vi "测量流程.vi"(11 "控制命令":T1(ring)) -> ()   [LabVIEW 2016, in "斯坦道氨氮.lvlib"]
uses:
  <vilib>/ptbypt/NI_PtbyPt.lvlib
panel:
  out "x-y":dbl
  out "当前时间":timestamp
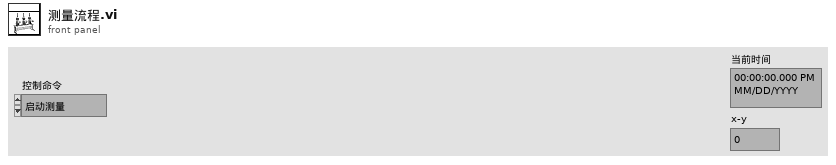
[diagram p1: front panel]
types:
  T1 = enum16{"启动测量", "标样核查", "零点核查", "跨度核查", "空白测试", "平行样测试", "加标回收", "空白校准", "标样校准", "初始化（清洗）", "停止测试", "仪器重启", "校时", "模式设置", "测量间隔设置"}
  T2 = cluster{"站号":u16, "量程切换":enum32{"H", "L", "AUTO"}, "控制命令":enum16{"启动测量", "标样核查", "零点核查", "跨度核查", "空白测试", "平行样测试", "加标回收", "空白校准", "标样校准", "初始化（清洗）", "停止测试", "仪器重启", "校时", "模式设置", "测量间隔设置"}, "模式设置":enum16{"待机", "连续模式", "周期模式", "定点模式", "受控模式", "手动模式"}, "测量间隔":u16}
  T3 = typedef "报警信息字段定义.ctl" = cluster{"时间":timestamp, "参数":string, "报警信息":string, "备注":string}
  T4 = cluster{"时间标识":timestamp, "设备":string, "日志信息":string, "流程参数":string}
  T5 = enum16{"空闲", "水样测试", "标样核查", "零点核查", "跨度核查", "空白测试", "平行样测试", "加标回收", "空白校准", "标样校准", "初始化（清洗）"}
  T6 = cluster{"系统时间":timestamp, "工作状态":u16, "测量模式":enum16{"待机", "连续模式", "周期模式", "定点模式", "受控模式", "手动模式"}, "告警代码":u16, "故障代码":u16, "日志代码":u16, "软件版本":u16, "F0":sgl, "F1":sgl, "F2":sgl, "F3":sgl, "T":sgl, "H":sgl, "id":u16, "flowid":u16, "量程":u16, "总磷控温温度1":sgl, "营养盐控温温度2":sgl, "ADC":sgl}
  T7 = cluster{"水样测试量程模式":enum16{"H", "L", "AUTO"}, "空白核查量程模式":enum16{"H", "L", "AUTO"}, "跨度核查量程模式":enum16{"H", "L", "AUTO"}, "加标回收量程模式":enum16{"H", "L", "AUTO"}, "标样核查量程模式":enum16{"H", "L", "AUTO"}}
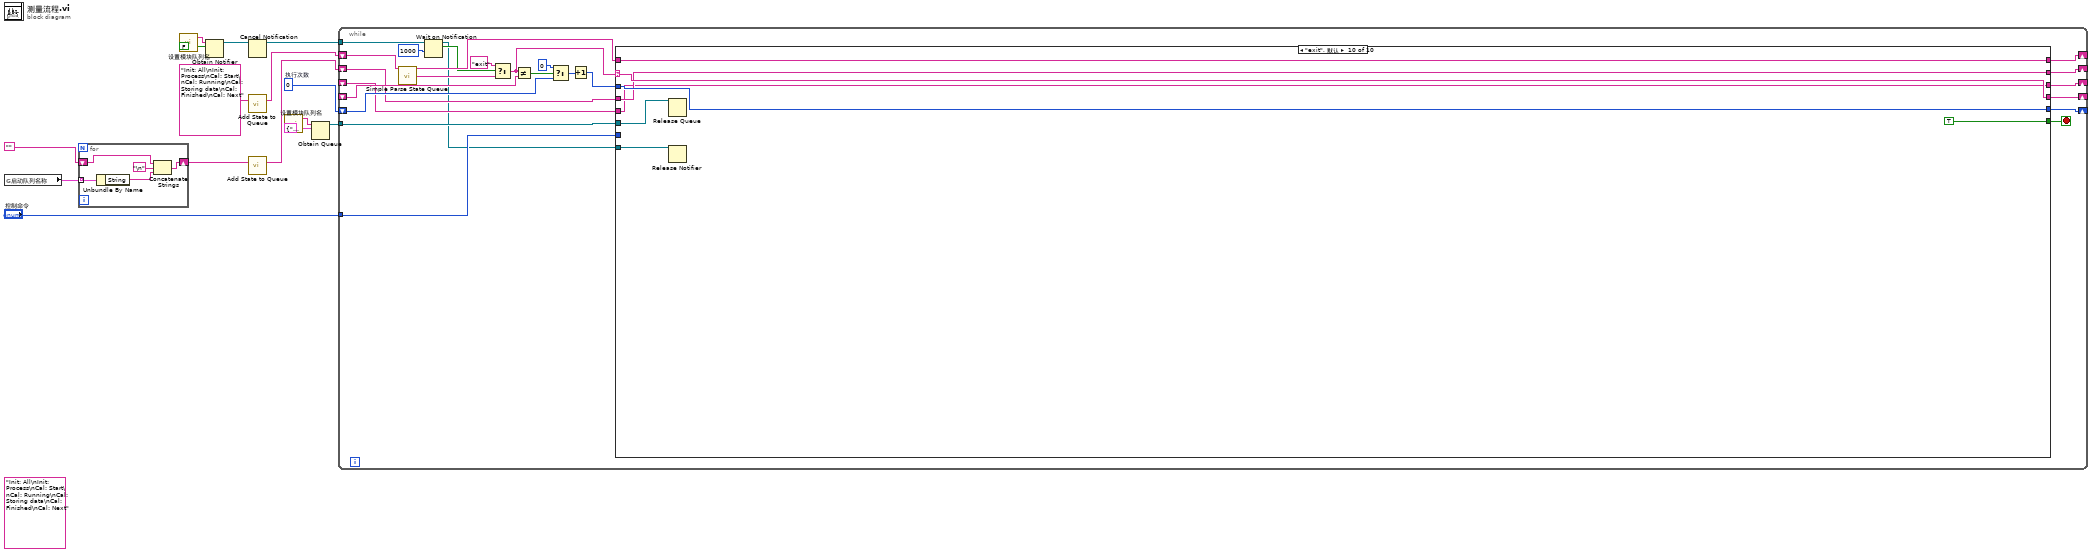
[diagram p0: block diagram]
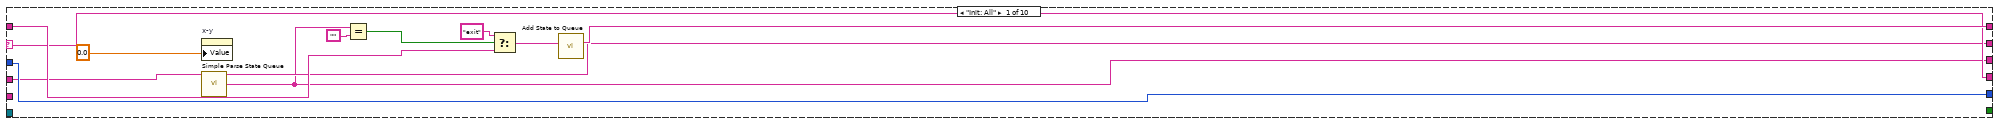
[diagram p2: hidden frame]
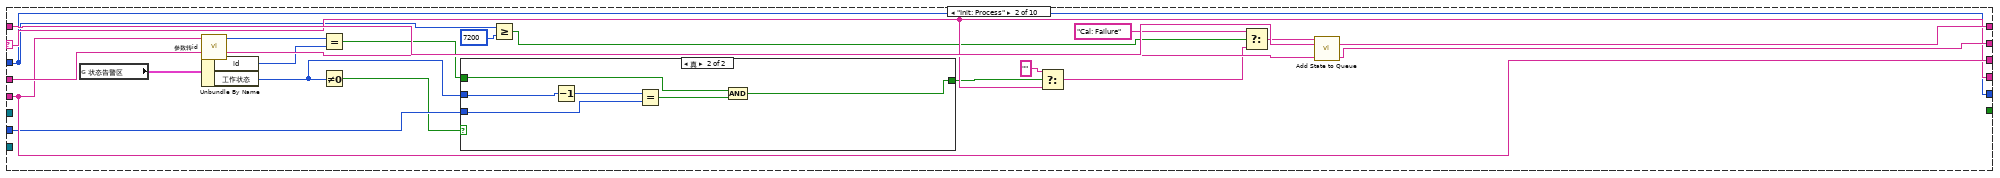
[diagram p3: hidden frame]
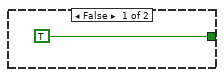
[diagram p4: hidden frame]
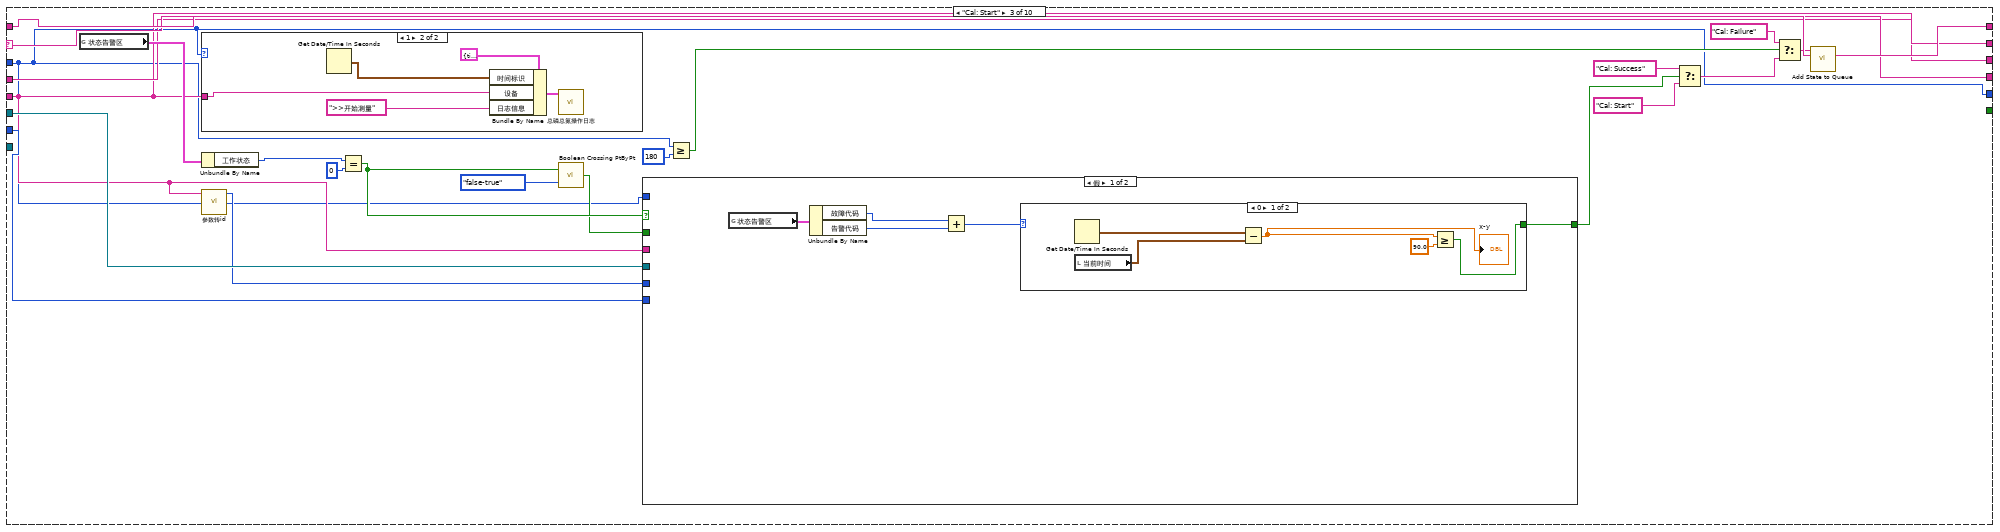
[diagram p5: hidden frame]
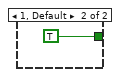
[diagram p6: hidden frame]
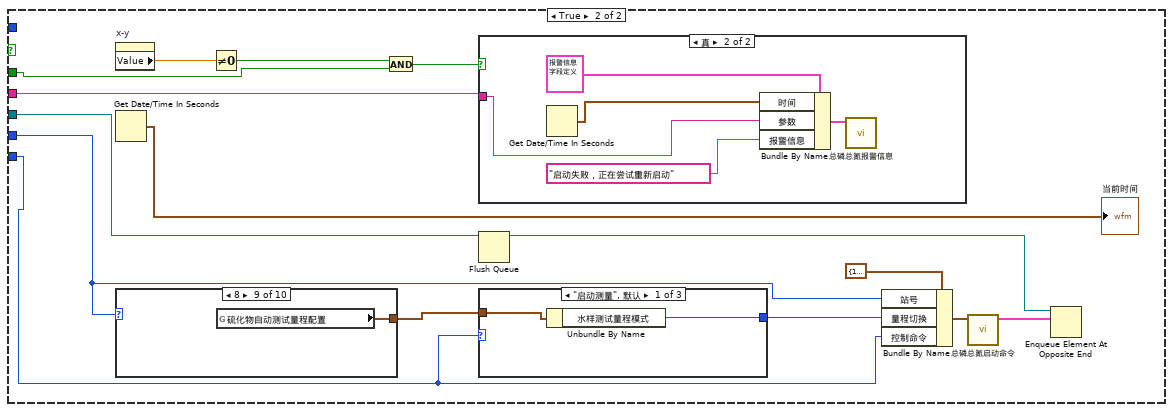
[diagram p7: hidden frame]
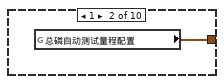
[diagram p10: hidden frame]
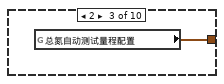
[diagram p11: hidden frame]
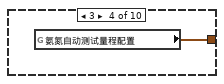
[diagram p12: hidden frame]
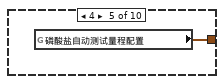
[diagram p13: hidden frame]
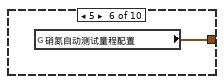
[diagram p14: hidden frame]
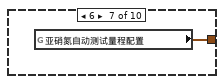
[diagram p15: hidden frame]
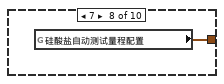
[diagram p16: hidden frame]
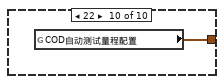
[diagram p17: hidden frame]
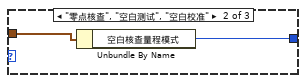
[diagram p18: hidden frame]
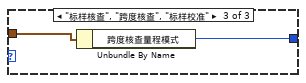
[diagram p19: hidden frame]
diagram:
  (unwired) "Init: All\nInit: Process\nCal: Start\nCal: Running\nCal: Storing data\nCal: Finished\nCal: Next" ("State(s) In (\"\")")
  w9 = 0  # 执行次数
  n1 = global read "model config var.vi" "启动队列名称"() -> (w1:cluster{"String":string, "Value":u16}[])
  n2 = for {
    shift-right: [w19] -> w2
    shift-left: "" -> [w20]
    tunnel: w1 -> [w18] mode=indexing
    n3 = Unbundle By Name(w18) -> ("String"=w17:string)
    n4 = Concatenate Strings(w20, "\n", w17) -> (w19:string)
  }
  n5 = call "设置模块队列名.vi"() -> ("Msg"=w6:string)  [unwired: 5 in]
  n6 = Obtain Notifier(name (unnamed)=w6, notification data type=FALSE) -> (notifier out=w14:refnum<notifier>)  [unwired: 2 in, 2 out]
  n7 = Cancel Notification(0:w14) -> (8:w4:refnum<notifier>)  [unwired: 1 in, 2 out]
  n8 = call "Add State to Queue.vi"("State(s) In (\"\")"="Init: All\nInit: Process\nCal: Start\nCal: Running\nCal: Storing data\nCal: Finished\nCal: Next" ("State(s) In (\"\")")) -> ("States Out"=w12:string)  [unwired: 14 in]
  n9 = call "Add State to Queue.vi"("State(s) In (\"\")"=w2) -> ("States Out"=w7:string)  [unwired: 14 in]
  n10 = call "设置模块队列名.vi"() -> ("Msg"=w5:string)  [unwired: 5 in]
  n11 = Obtain Queue(name (unnamed)=w5, element data type=cluster{"命令":string, "data":variant} {"命令"="", "data"=variant}) -> (queue out=w10:refnum<queue>)  [unwired: 3 in, 2 out]
  n12 = while {
    tunnel: w10 -> [w43]
    shift-right: [w42] -> _
    shift-left: w12 -> [w45]
    shift-right: [w35] -> _
    shift-left: w9 -> [w38]
    shift-right: [w41] -> _
    shift-left: _ -> [w40]
    tunnel: "控制命令" -> [w33]
    shift-right: [w29] -> _
    shift-left: w7 -> [w31]
    shift-right: [w30] -> _
    shift-left: _ -> [w28]
    tunnel: w4 -> [w26]
    stop <- w32 stop-if-true
    n13 = call "Simple Parse State Queue.vi"("State Queue"=w45) -> ("Remain States"=w44:string, "Next State"=w23:string)  [unwired: 13 in]
    n14 = Wait on Notification(notifier=w26, timeout in ms (-1)=1000 ("超时毫秒(-1)")) -> (notifier out=w21:refnum<notifier>, notification=w25:bool)  [unwired: 2 in, 2 out]
    n15 = Select(t="exit", s=w25, f=w23) -> (s? t:f=w22:string)
    n16 = Not Equal?(x=w22, y=w40) -> (x != y?=w39:bool)
    n17 = Select(t=0, s=w39, f=w38) -> (s? t:f=w36:i32)
    n18 = Increment(x=w36) -> (x+1=w34:i32)
    n19 = case shown="\"exit\", 默认" w22 {
      selector: w22 -> [w53 w66 w105 w162 w177 w183 w197 w213 w224 w231]
      tunnel: w44 -> [w55 w76 w107 w164 _ w194 w202 w215 _ w232]
      tunnel: w43 -> [_ _ w103 _ _ _ _ _ _ w227]
      tunnel: [w57 w77 w106 w163 w178 w193 w201 w214 "Init: All\nInit: Process\nCal: Start\nCal: Running\nCal: Storing data\nCal: Finished\nCal: Next" ("State(s) In (\"\")") w232] -> w42
      tunnel: [w53 w66 w105 w162 w177 w183 w197 w213 w224 w231] -> w41
      tunnel: [w52 w65 w85 w161 w176 w186 w200 w211 w223 w230] -> w35
      tunnel: w34 -> [w52 w65 w85 w161 w176 w186 w200 w211 w223 w230]
      tunnel: w33 -> [_ w70 w102 _ _ _ _ _ _ _]
      tunnel: [_ _ _ _ _ _ _ _ _ TRUE] -> w32
      tunnel: w31 -> [w51 w75 w93 w160 w170 w180 w204 w212 w222 w229]
      tunnel: [w49 w73 w87 w159 w169 w179 w203 w210 w221 w228] -> w30
      tunnel: [w50 w75 w93 w160 w170 w180 w204 w212 w222 w229] -> w29
      tunnel: w28 -> [_ w73 w87 w159 w169 w179 w203 w210 w221 w228]
      tunnel: w21 -> [_ _ _ _ _ _ _ _ _ w226]
      frame "Init: All" {
        n20 = property on="x-y" class="DigNum (严格)"("Value"=0.0 ("x-y")) -> ()  [unwired: 2 in, 2 out]
        n21 = call "Simple Parse State Queue.vi"("State Queue"=w51) -> ("Remain States"=w50:string, "Next State"=w49:string)  [unwired: 13 in]
        n22 = Equal?(x=w49, y="") -> (x = y?=w47:bool)
        n23 = Select(t="exit", s=w47, f=w55) -> (s? t:f=w54:string)
        n24 = call "Add State to Queue.vi"("State(s) In (\"\")"=w54) -> ("States Out"=w57:string)  [unwired: 14 in]
      }
      frame "Init: Process" {
        n25 = global read "VAR总磷总氮全局变量.vi" "状态告警区"() -> (w74:T6)
        n26 = call "参数转id.vi"("table"=w73) -> ("id"=w71:u16)  [unwired: 10 in]
        n27 = Unbundle By Name(w74) -> ("id"=w72:u16, "工作状态"=w68:u16)
        n28 = Equal?(x=w71, y=w72) -> (x = y?=w59:bool)
        n29 = Not Equal To 0?(x=w68) -> (x != 0?=w69:bool)
        n30 = case shown="真" w69 {
          tunnel: w68 -> [_ w84]
          tunnel: w70 -> [_ w82]
          tunnel: [TRUE w79] -> w58
          tunnel: w59 -> [_ w80]
          frame False {
          }
          frame True {
            n31 = Decrement(x=w84) -> (x-1=w83:u16)
            n32 = Equal?(x=w83, y=w82) -> (x = y?=w81:bool)
            n33 = And(x=w80, y=w81) -> (x .and. y?=w79:bool)
          }
        }
        n34 = Greater Or Equal?(x=w65, y=7200) -> (x >= y?=w63:bool)
        n35 = Select(t="", s=w58, f=w66) -> (s? t:f=w61:string)
        n36 = Select(t="Cal: Failure", s=w63, f=w61) -> (s? t:f=w60:string)
        n37 = call "Add State to Queue.vi"("State(s) In Front (\"\")"=w60, "State(s) In (\"\")"=w76) -> ("States Out"=w77:string)  [unwired: 13 in]
      }
      frame "Cal: Start" {
        n38 = global read "VAR总磷总氮全局变量.vi" "状态告警区"() -> (w104:T6)
        n39 = case shown="1" w85 {
          tunnel: w87 -> [_ w154]
          frame 0, Default {
          }
          frame 1 {
            n40 = Get Date/Time In Seconds() -> (seconds since 1Jan1904=w158:timestamp)
            n41 = Bundle By Name(cluster=T4 {"时间标识"=timestamp(0 s since 1904-01-01), "设备"="", "日志信息"="", "流程参数"=""} ("data in"), "时间标识"=w158, "设备"=w154, "日志信息"=">>开始测量") -> (w157:T4)
            n42 = call "总磷总氮操作日志.vi"("data in"=w157) -> ()  [unwired: 10 in, 1 out]
          }
        }
        n43 = Unbundle By Name(w104) -> ("工作状态"=w92:u16)
        n44 = call "参数转id.vi"("table"=w87) -> ("id"=w86:u16)  [unwired: 10 in]
        n45 = Equal?(x=w92, y=u16 0) -> (x = y?=w90:bool)
        n46 = call <vilib>:"Boolean Crossing PtByPt.vi"("direction"=enum16{"either", "false-true", "true-false"}."false-true", "input"=w90) -> ("crossing"=w88:bool)  [unwired: 1 in]
        n47 = case shown="假" w90 {
          tunnel: w102 -> [_ w129]
          tunnel: w103 -> [_ w132]
          tunnel: [w112 _] -> w97
          tunnel: w86 -> [_ w127]
          tunnel: w85 -> [_ _]
          tunnel: w87 -> [_ w121]
          tunnel: w88 -> [_ w119]
          frame False {
            n48 = global read "VAR总磷总氮全局变量.vi" "状态告警区"() -> (w111:T6)
            n49 = Unbundle By Name(w111) -> ("故障代码"=w109:u16, "告警代码"=w110:u16)
            n50 = Add(x=w109, y=w110) -> (x+y=w108:u16)
            n51 = case shown="0" w108 {
              tunnel: [w113 TRUE] -> w112
              frame 0 {
                n52 = Get Date/Time In Seconds() -> (seconds since 1Jan1904=w116:timestamp)
                n53 = local read "当前时间"() -> (w117:timestamp)
                n54 = Subtract(x=w116, y=w117) -> (x-y=w115:dbl)
                "x-y" <- w115
                n55 = Greater Or Equal?(x=w115, y=90.0) -> (x >= y?=w113:bool)
              }
              frame 1, Default {
              }
            }
          }
          frame True {
            n56 = property on="x-y" class="DigNum (严格)"() -> ("Value"=w123:dbl)  [unwired: 2 in, 2 out]
            n57 = Get Date/Time In Seconds() -> (seconds since 1Jan1904=→"当前时间":timestamp)
            n58 = case shown="8" w127 {
              tunnel: [_ w139 w140 w141 w142 w143 w144 w145 w146 w147] -> w128
              frame 0, Default {
              }
              frame 1 {
                n59 = global read "总磷总氮断电保存全局变量.vi" "总磷自动测试量程配置"() -> (w139:T7)
              }
              frame 2 {
                n60 = global read "总磷总氮断电保存全局变量.vi" "总氮自动测试量程配置"() -> (w140:T7)
              }
              frame 3 {
                n61 = global read "总磷总氮断电保存全局变量.vi" "氨氮自动测试量程配置"() -> (w141:T7)
              }
              frame 4 {
                n62 = global read "总磷总氮断电保存全局变量.vi" "磷酸盐自动测试量程配置"() -> (w142:T7)
              }
              frame 5 {
                n63 = global read "总磷总氮断电保存全局变量.vi" "硝氮自动测试量程配置"() -> (w143:T7)
              }
              frame 6 {
                n64 = global read "总磷总氮断电保存全局变量.vi" "亚硝氮自动测试量程配置"() -> (w144:T7)
              }
              frame 7 {
                n65 = global read "总磷总氮断电保存全局变量.vi" "硅酸盐自动测试量程配置"() -> (w145:T7)
              }
              frame 8 {
                n66 = global read "总磷总氮断电保存全局变量.vi" "硫化物自动测试量程配置"() -> (w146:T7)
              }
              frame 22 {
                n67 = global read "总磷总氮断电保存全局变量.vi" "COD自动测试量程配置"() -> (w147:T7)
              }
            }
            n68 = Not Equal To 0?(x=w123) -> (x != 0?=w122:bool)
            n69 = And(x=w122, y=w119) -> (x .and. y?=w120:bool)
            n70 = case shown="真" w120 {
              tunnel: w121 -> [_ w136]
              frame False {
              }
              frame True {
                n71 = Get Date/Time In Seconds() -> (seconds since 1Jan1904=w135:timestamp)
                n72 = Bundle By Name(cluster=T3 {"时间"=timestamp(0 s since 1904-01-01), "参数"="", "报警信息"="", "备注"=""} ("data in"), "时间"=w135, "参数"=w136, "报警信息"="启动失败，正在尝试重新启动") -> (w137:T3)
                n73 = call "总磷总氮报警信息.vi"("data in"=w137) -> ()  [unwired: 10 in, 1 out]
              }
            }
            n74 = Flush Queue(queue=w132) -> (queue out=w125:refnum<queue>)  [unwired: 1 in, 2 out]
            n75 = case shown="\"启动测量\", 默认" w129 {
              tunnel: w128 -> [w149 w151 w153]
              tunnel: [w148 w150 w152] -> w133
              frame "启动测量", Default {
                n76 = Unbundle By Name(w149) -> ("水样测试量程模式"=w148:enum16{"H", "L", "AUTO"})
              }
              frame "零点核查", "空白测试", "空白校准" {
                n77 = Unbundle By Name(w151) -> ("空白核查量程模式"=w150:enum16{"H", "L", "AUTO"})
              }
              frame "标样核查", "跨度核查", "标样校准" {
                n78 = Unbundle By Name(w153) -> ("跨度核查量程模式"=w152:enum16{"H", "L", "AUTO"})
              }
            }
            n79 = Bundle By Name(cluster=T2 {"站号"=1, "量程切换"=enum."AUTO", "控制命令"=enum."启动测量", "模式设置"=enum."待机", "测量间隔"=0} ("参数"), "站号"=w127, "量程切换"=w133, "控制命令"=w129) -> (w130:T2)
            n80 = call "总磷总氮启动命令.vi"("参数"=w130) -> ("启动命令"=w126:cluster{"命令":string, "data":variant})  [unwired: 10 in]
            n81 = Enqueue Element At Opposite End(queue=w125, element=w126) -> ()  [unwired: 2 in, 3 out]
          }
        }
        n82 = Greater Or Equal?(x=w85, y=180) -> (x >= y?=w100:bool)
        n83 = Select(t="Cal: Success" ("State(s) In (\"\")"), s=w97, f="Cal: Start" ("State(s) In (\"\")")) -> (s? t:f=w95:string)
        n84 = Select(t="Cal: Failure" ("State(s) In (\"\")"), s=w100, f=w95) -> (s? t:f=w98:string)
        n85 = call "Add State to Queue.vi"("State(s) In Front (\"\")"=w98, "State(s) In (\"\")"=w107) -> ("States Out"=w106:string)  [unwired: 13 in]
      }
      frame "Cal: Success" {
        n86 = Get Date/Time In Seconds() -> (seconds since 1Jan1904=w167:timestamp)
        n87 = Bundle By Name(cluster=T4 {"时间标识"=timestamp(0 s since 1904-01-01), "设备"="", "日志信息"="", "流程参数"=""} ("data in"), "时间标识"=w167, "设备"=w159, "日志信息"="-->>启动成功") -> (w166:T4)
        n88 = call "总磷总氮操作日志.vi"("data in"=w166) -> ()  [unwired: 10 in, 1 out]
        n89 = call "Add State to Queue.vi"("State(s) In (\"\")"=w164) -> ("States Out"=w163:string)  [unwired: 14 in]
      }
      frame "Cal: Failure" {
        n90 = Get Date/Time In Seconds() -> (seconds since 1Jan1904=w174:timestamp)
        n91 = Bundle By Name(cluster=T4 {"时间标识"=timestamp(0 s since 1904-01-01), "设备"="", "日志信息"="", "流程参数"=""} ("data in"), "时间标识"=w174, "设备"=w169, "日志信息"="-->>启动失败") -> (w173:T4)
        n92 = call "总磷总氮操作日志.vi"("data in"=w173) -> ()  [unwired: 10 in, 1 out]
        n93 = call "Add State to Queue.vi"("State(s) In (\"\")"="exit" ("State(s) In (\"\")")) -> ("States Out"=w178:string)  [unwired: 14 in]
      }
      frame "Cal: Running" {
        n94 = global read "VAR总磷总氮全局变量.vi" "状态告警区"() -> (w190:T6)
        n95 = Unbundle By Name(w190) -> ("工作状态"=w191:u16)
        n96 = Less Or Equal?(x=w186, y=7200) -> (x <= y?=w184:bool)
        n97 = Select(t=w183, s=w184, f="exit") -> (s? t:f=w182:string)
        n98 = Equal?(x=w191, y=T5."空闲") -> (x = y?=w189:bool)
        n99 = Select(t="", s=w189, f=w182) -> (s? t:f=w187:string)
        n100 = call "Add State to Queue.vi"("State(s) In Front (\"\")"=w187, "State(s) In (\"\")"=w194) -> ("States Out"=w193:string)  [unwired: 13 in]
      }
      frame "Cal: Storing data" {
        n101 = case shown="1" w200 {
          tunnel: w203 -> [_ w205]
          frame 0, Default {
          }
          frame 1 {
            n102 = Get Date/Time In Seconds() -> (seconds since 1Jan1904=w209:timestamp)
            n103 = Bundle By Name(cluster=T4 {"时间标识"=timestamp(0 s since 1904-01-01), "设备"="", "日志信息"="", "流程参数"=""} ("data in"), "时间标识"=w209, "设备"=w205, "日志信息"="-->>存储数据") -> (w208:T4)
            n104 = call "总磷总氮操作日志.vi"("data in"=w208) -> ()  [unwired: 10 in, 1 out]
          }
        }
        n105 = Less Or Equal?(x=w200, y=60) -> (x <= y?=w198:bool)
        n106 = Select(t=w197, s=w198, f="") -> (s? t:f=w195:string)
        n107 = call "Add State to Queue.vi"("State(s) In Front (\"\")"=w195, "State(s) In (\"\")"=w202) -> ("States Out"=w201:string)  [unwired: 13 in]
      }
      frame "Cal: Finished" {
        n108 = case shown="1" w211 {
          tunnel: w210 -> [_ w216]
          frame 0, Default {
          }
          frame 1 {
            n109 = Get Date/Time In Seconds() -> (seconds since 1Jan1904=w220:timestamp)
            n110 = Bundle By Name(cluster=T4 {"时间标识"=timestamp(0 s since 1904-01-01), "设备"="", "日志信息"="", "流程参数"=""} ("data in"), "时间标识"=w220, "设备"=w216, "日志信息"="测量结束>>") -> (w219:T4)
            n111 = call "总磷总氮操作日志.vi"("data in"=w219) -> ()  [unwired: 10 in, 1 out]
          }
        }
        n112 = call "Add State to Queue.vi"("State(s) In (\"\")"=w215) -> ("States Out"=w214:string)  [unwired: 14 in]
      }
      frame "Cal: Next" {
      }
      frame "exit", Default {
        n113 = Release Queue(queue=w227) -> ()  [unwired: 2 in, 3 out]
        n114 = Release Notifier(notifier=w226) -> ()  [unwired: 2 in, 3 out]
      }
    }
  }
